vi "Parser_0x54_(SubVI).vi"(11 "String in":string) -> (3 "Номер табличного параметра":i32, 5 "CheckSumGood":bool)   [LabVIEW 2017, in "LV_Unicorn.lvlib"]
uses:
  LV_Unicorn.lvlib
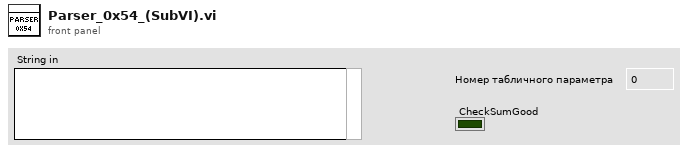
[diagram p1: front panel]
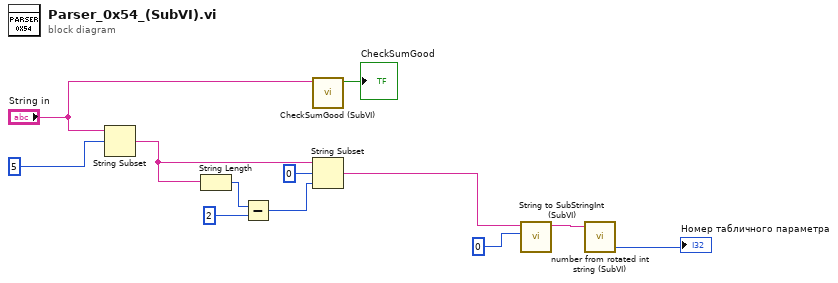
[diagram p0: block diagram]
diagram:
  n1 = String Subset(string="String in", offset (0)=5) -> (substring=w3:string)  [unwired: 1 in]
  n2 = String Length(string=w3) -> (length=w8:i32)
  n3 = Subtract(x=w8, y=2) -> (x-y=w4:i32)
  n4 = call "CheckSumGood (SubVI).vi"("String in"="String in") -> ("CheckSumGood"=→"CheckSumGood":bool)  [unwired: 10 in]
  n5 = String Subset(string=w3, offset (0)=0, length (rest)=w4) -> (substring=w5:string)
  n6 = call "String to SubStringInt (SubVI).vi"("Nx4byte"=u32 0, "String in in"=w5) -> ("String out"=w10:string)  [unwired: 9 in]
  n7 = call "number from rotated int string (SubVI).vi"("String"=w10) -> ("int number"=→"Номер табличного параметра":i32)  [unwired: 2 in, 2 out]
